vi "Pulse Measurement Panel.vi"(0 "RFmx Settings":T1={"Center Frequency (Hz)"=10000000000.0, "Measurement Bandwidth (Hz)"=80000000.0, "Reference Level (dBm)"=10.0, "RFmx De-embedding"={"RFmx Name"="5842_0", "RFmx Port"="", "Attenuation"={"Mode"=enum."Constant Attenuation", "Constant Attenuation"={"RFmx External Attenuation (dB)"=1.2}, "s2p File"={"RFmx S-Parameters Orientation"=24000, "RFmx Attenuation s2p Path Name"="", "RFmx Attenuation s2p File"=path ""}}}, "Acquisition Length (s)"=0.0} {"RFmx De-embedding"."Attenuation"."s2p File"."RFmx S-Parameters Orientation" items=["Port1 Towards DUT"=24000, "Port2 Towards DUT"=24001]; "RFmx De-embedding"."Attenuation"."Constant Attenuation"."RFmx External Attenuation (dB)" format="%.2f"; "Reference Level (dBm)" format="%.2f"; "Measurement Bandwidth (Hz)" format="%.3p"; "Center Frequency (Hz)" format="%.6p"}, 5 "RFSG settings":T3={"RFSG De-embedding"={"RFSG Name"="5842_0", "RFSG Port"="", "Attenuation"={"Mode"=enum."Constant Attenuation", "Contant Attenuation"={"RFSG External Attenuation (dB)"=2.0}, "s2p File"={"RFSG S-parameters Orientation"=24000, "RFSG Attenuation s2p Path Name"="", "RFSG s2p File Path"=path ""}}}, "Generation IQ Rate (S/s)"=0.0} {"RFSG De-embedding"."Attenuation"."s2p File"."RFSG S-parameters Orientation" items=["Port1 Towards DUT"=24000, "Port2 Towards DUT"=24001]; "RFSG De-embedding"."Attenuation"."Contant Attenuation"."RFSG External Attenuation (dB)" format="%.2f"}, 7 "Test Configuration":T5, 11 "error in":errorcluster) -> (3 "Per Pulse Results (Header Name)":string[](array[string]), 4 "TS Intrapulse Stability":dbl[][](array[numeric]), 6 "TS P2P Stability":dbl[][](array[numeric]), 8 "Per Pulse Results (for MP)":dbl[][](array[numeric])=[[-60.19434452056885, -48.23559761047363, -61.500163078308105, -61.676697731018066, -50.09932041168213, -61.2670373916626, -47.940940856933594, -60.594682693481445, -54.222588539123535, -68.17487716674805], [-51.47902011871338, -63.676371574401855, -49.32386875152588, -42.60602951049805, -41.78941249847412, -56.57611846923828, -67.04894065856934, -44.43309783935547, -53.89562129974365, -45.59821605682373], [-50.93127727508545, -48.11325550079346, -49.06841278076172, -42.55256652832031, -41.191606521606445, -55.30652046203613, -47.88793087005615, -44.32924270629883, -51.04572772979736, -45.574283599853516], [0.7774313706217917, 0.7743052754564207, 0.6733820768651879, 0.6972024148638998, 0.6739289285829677, 0.8012453172128895, 0.7789831746751243, 0.81331101938709, 0.6993593760935255, 0.7751122603266651], [-0.04818759954671978, -0.17045354969029822, -0.2937592841444876, -0.18006245433349588, -0.30206692305208827, -0.23840372056041464, -0.22733917807886903, -0.2726908323785403, -0.20409866605988866, -0.22706977878895118], [1.8971785430084185, 1.7078184861447125, 1.6125145446758244, 1.6429880662265446, 1.7003339064410368, 1.645767369340552, 1.8225724908268657, 1.500202053052531, 1.816586601520762, 1.7434164608706486], [9.902169056670972e-09, 1.0171003831640633e-08, 1.0087378671871648e-08, 1.0018839745468426e-08, 1.0021453073999283e-08, 9.937162678335199e-09, 1.0113660404718986e-08, 9.936247799288367e-09, 1.0029181489475149e-08, 1.0014254033422958e-08], [1.1747647026741224e-08, 0.00010001147191839247, 0.00020001407632828564, 0.0003000116995963527, 0.00040001415077715896, 0.0005000116894758734, 0.0006000140392077577, 0.000700011761394561, 0.0008000141195439436, 0.000900014054837663], [1.0266075038352937e-08, 1.0210194009332553e-08, 9.96602777140197e-09, 1.0195131948175912e-08, 1.0214687343427613e-08, 1.0248380139892106e-08, 1.003600972591812e-08, 1.0209683835273609e-08, 1.0208458229471944e-08, 1.0051256216333969e-08], [2.0016060941649103e-05, 0.00012001605265167608, 0.0002200186251165217, 0.0003200161244125173, 0.00042001858918951285, 0.0005200161200707459, 0.000620018587380489, 0.0007200160772447398, 0.0008200186061427676, 0.0009200186490169424], [1.9999915173664064e-05, 1.9999928162649538e-05, 1.9999979315091006e-05, 1.9999962883326592e-05, 1.9999940266618827e-05, 1.9999970715330443e-05, 1.9999948164994597e-05, 1.999989449659788e-05, 1.9999961878396942e-05, 2.0000044728873845e-05], [8.000006128542082e-05, 8.000009557087724e-05, 8.000003688745302e-05, 8.000002009960112e-05, 8.000005863752275e-05, 8.000001971001538e-05, 8.000010310677254e-05, 8.000006664992009e-05, 8.000000105017845e-05, nan], [19.999919881828227, 19.999923415962357, 19.999976074586076, 19.99996628673531, 19.99994048578986, 19.999972630258657, 19.999937910673005, 19.999902267256314, 19.99996929267048, nan], [9.999997645908488e-05, 0.00010000002373352679, 0.00010000001620254403, 9.999998298292771e-05, 9.999999890414157e-05, 9.999999042534582e-05, 0.00010000005127176714, 9.999996114651797e-05, 9.99999629285754e-05, nan]], 10 "TS Acquired Amplitude":dbl[][](array[numeric]), 15 "error out":errorcluster)   [LabVIEW 2023]
doc: "This example demonstrates the configuration of Pulse signal basic properties for measuring the stability properties of a pulse. This example enables traces to view the time domain stability and Pulse to Pulse Stability Traces ."
uses:
  Controls/RFmx Config - Pulse.ctl
  FPT Shared VIs/De-embedding/RFmx Config.ctl
  Controls/RFSG Config - Pulse.ctl
  FPT Shared VIs/De-embedding/RFsg Config.ctl
  Controls/Test Config - Pulse.ctl
panel:
  in  "Stop":bool
  in  "Configuration Tabs":enum32{"RFmx", "RFSG", "Test Configuration"}(tab)
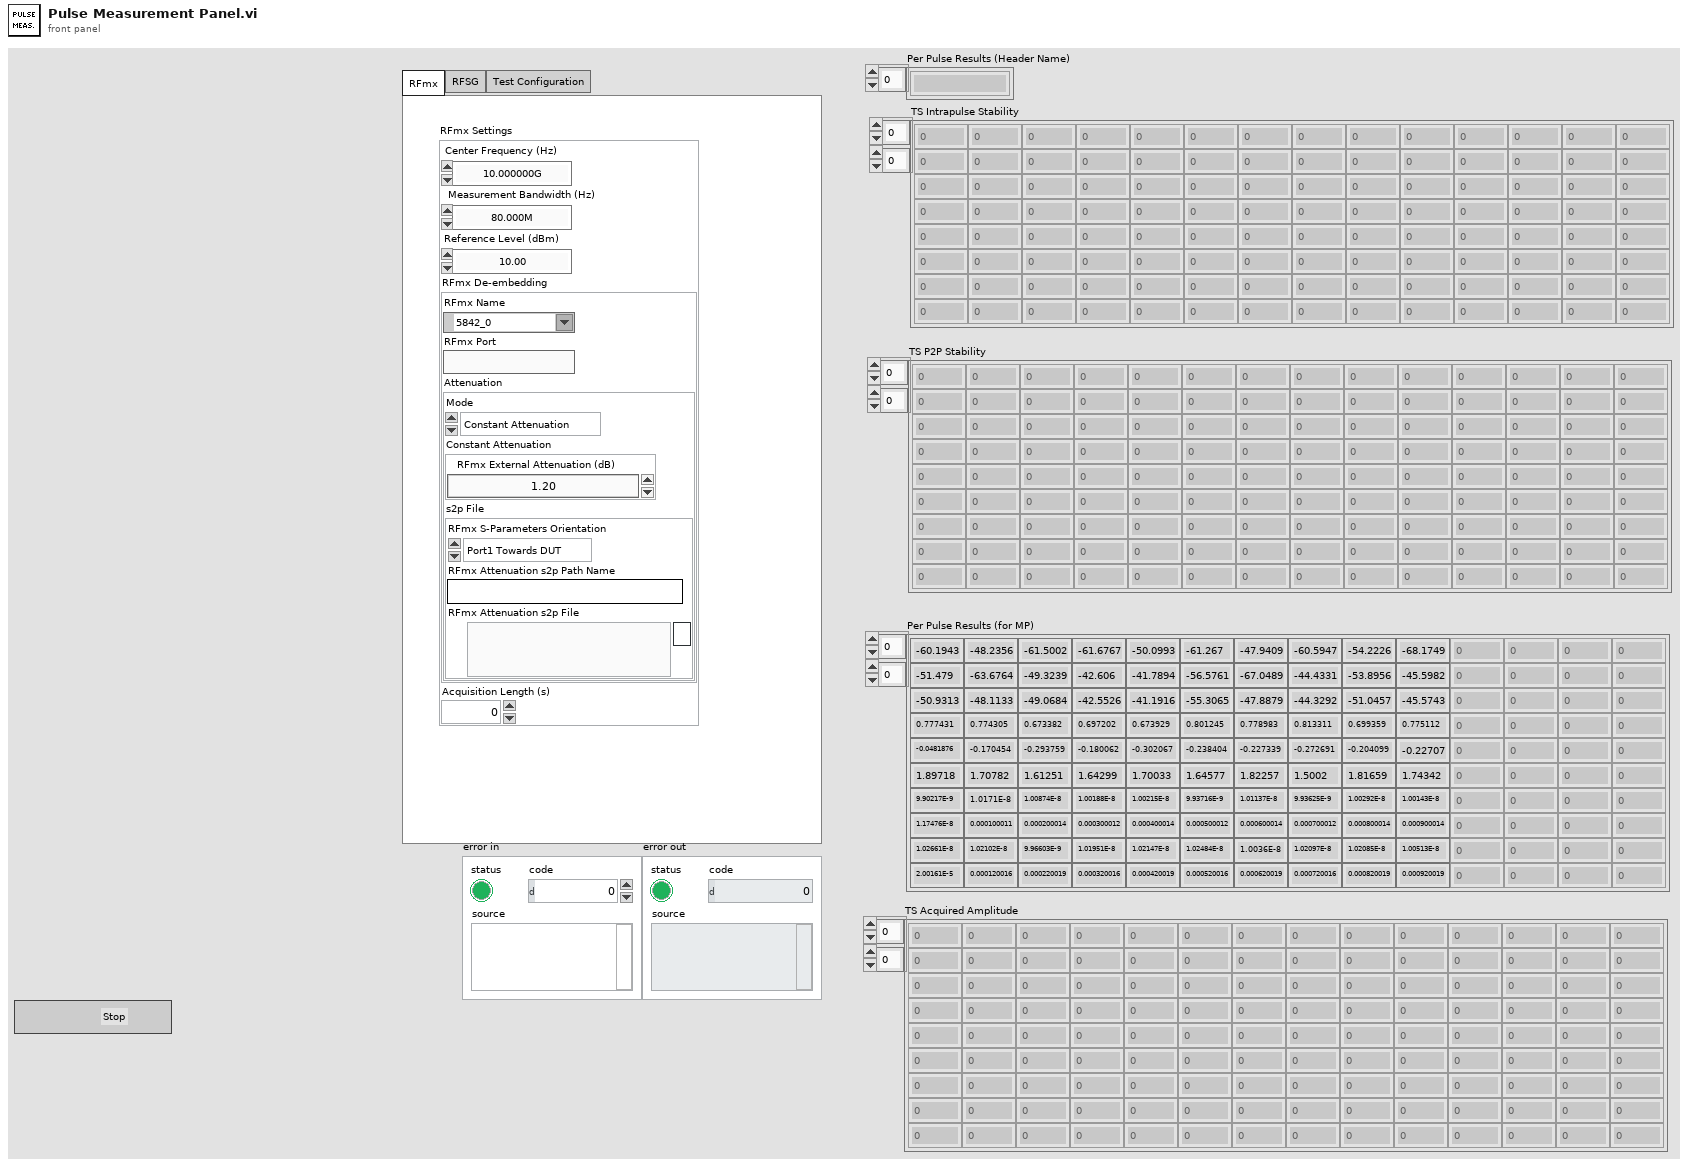
[diagram p1: front panel]
types:
  T1 = typedef "RFmx Config - Pulse.ctl" = cluster{"Center Frequency (Hz)":dbl, "Measurement Bandwidth (Hz)":dbl, "Reference Level (dBm)":dbl, "RFmx De-embedding":T2, "Acquisition Length (s)":dbl}
  T2 = typedef "RFmx Config.ctl" = cluster{"RFmx Name":refnum<k15>, "RFmx Port":string, "Attenuation":cluster{"Mode":enum32{"<None>", "Constant Attenuation", "s2p File"}, "Constant Attenuation":cluster{"RFmx External Attenuation (dB)":dbl}, "s2p File":cluster{"RFmx S-Parameters Orientation":i32, "RFmx Attenuation s2p Path Name":string, "RFmx Attenuation s2p File":path}}}
  T3 = typedef "RFSG Config - Pulse.ctl" = cluster{"RFSG De-embedding":T4, "Generation IQ Rate (S/s)":dbl}
  T4 = typedef "RFsg Config.ctl" = cluster{"RFSG Name":refnum<k15>, "RFSG Port":string, "Attenuation":cluster{"Mode":enum32{"<None>", "Constant Attenuation", "s2p File"}, "Contant Attenuation":cluster{"RFSG External Attenuation (dB)":dbl}, "s2p File":cluster{"RFSG S-parameters Orientation":i32, "RFSG Attenuation s2p Path Name":string, "RFSG s2p File Path":path}}}
  T5 = typedef "Test Config - Pulse.ctl" = cluster{"Pulse Configuration":cluster{"Power Level (dBm)":dbl, "Pulse Repetition Interval [PRI] (s)":dbl, "Pulse Width (s)":dbl, "Number of Pulses per Burst":u32}, "Pulse Stability":cluster{"Pulse Stability Meas Offset":i32, "Window Start (%)":dbl, "Window Stop (%)":dbl, "Window Step Size (%)":dbl, "Selected Pulse Trace":i32}, "Pulse Profile":cluster{"High Reference Level (%)":dbl, "Width Reference Level (%)":dbl, "Low Reference Level (%)":dbl}}
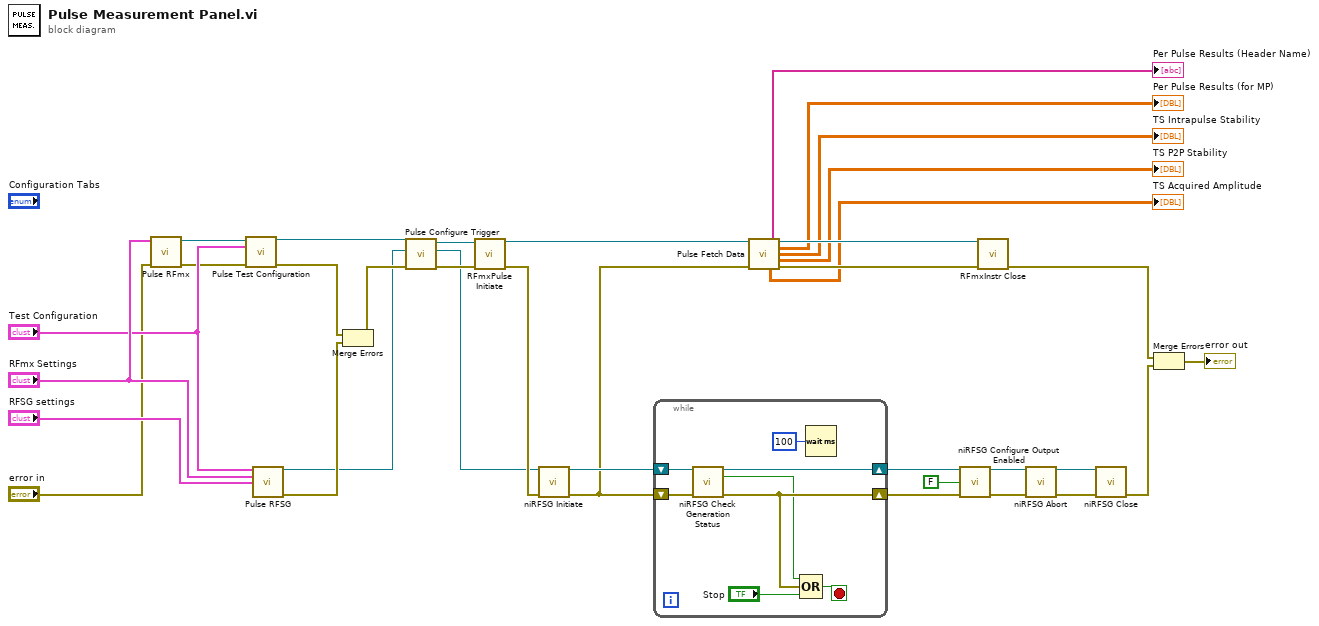
[diagram p0: block diagram]
diagram:
  n1 = call "Pulse RFmx.vi"("error in"="error in", "RFmx Settings"="RFmx Settings") -> ("error out"=w6:errorcluster, "RFmx session out"=w18:refnum<k21>)  [unwired: 8 in]
  n2 = call "Pulse Test Configuration.vi"("RFmx session in"=w18, "Test Configuration"="Test Configuration", "error in"=w6) -> ("RFmx session out"=w4:refnum<k21>, "error out"=w19:errorcluster)  [unwired: 11 in]
  n3 = call "Pulse RFSG.vi"("Test Configuration"="Test Configuration", "RFmx Settings"="RFmx Settings", "RFSG settings"="RFSG settings") -> ("RFSG session"=w2:refnum<k15>, "error out"=w20:errorcluster)  [unwired: 11 in]
  n4 = Merge Errors(w19, w20) -> (w24:errorcluster)
  n5 = call "Pulse Configure Trigger.vi"("error in"=w24, "RFSG session in"=w2, "RFmx session in"=w4) -> ("error out"=w5:errorcluster, "RFSG session out"=w1:refnum<k15>, "RFmx session out"=w3:refnum<k21>)  [unwired: 6 in]
  n6 = call <vilib>:"RFmxPulse Initiate.vi"("Instrument Handle In"=w3, "error in (no error)"=w5) -> ("Instrument Handle Out"=w33:refnum<k21>, "error out"=w28:errorcluster)  [unwired: 11 in, 1 out]
  n7 = call <instrlib>:"niRFSG Initiate.vi"("instrument handle"=w1, "error in"=w28) -> ("instrument handle out"=w32:refnum<k15>, "error out"=w27:errorcluster)  [unwired: 12 in]
  n8 = while {
    shift-right: [w42] -> w30
    shift-left: w32 -> [w43]
    shift-right: [w37] -> w29
    shift-left: w27 -> [w38]
    stop <- w41 stop-if-true
    n9 = call <instrlib>:"niRFSG Check Generation Status.vi"("instrument handle"=w43, "error in"=w38) -> ("instrument handle out"=w42:refnum<k15>, "done?"=w36:bool, "error out"=w37:errorcluster)  [unwired: 11 in]
    n10 = Compound Arithmetic op=OR(w36, w37, "Stop") -> (w41:bool)
    n11 = Wait (ms)(milliseconds to wait=u32 100) -> ()  [unwired: 1 out]
  }
  n12 = call "Pulse Fetch Data.vi"("RFmx Session in"=w33, "error in"=w27) -> ("Per Pulse Results (Header Name)"=→"Per Pulse Results (Header Name)":string[], "RFmx Session Out"=w35:refnum<k21>, "Per Pulse Results (for MP)"=→"Per Pulse Results (for MP)":dbl[][], "TS Intrapulse Stability"=→"TS Intrapulse Stability":dbl[][], "TS P2P Stability"=→"TS P2P Stability":dbl[][], "TS Acquired Amplitude"=→"TS Acquired Amplitude":dbl[][], "error out"=w34:errorcluster)  [unwired: 7 in]
  n13 = call <instrlib>:"niRFSG Configure Output Enabled.vi"("instrument handle"=w30, "output enabled"=FALSE ("output enable"), "error in"=w29) -> ("instrument handle out"=w22:refnum<k15>, "error out"=w21:errorcluster)  [unwired: 11 in]
  n14 = call <vilib>:"RFmxInstr Close.vi"("Instrument Handle In"=w35, "error in (no error)"=w34) -> ("error out"=w25:errorcluster)  [unwired: 13 in]
  n15 = call <instrlib>:"niRFSG Abort.vi"("instrument handle"=w22, "error in"=w21) -> ("instrument handle out"=w8:refnum<k15>, "error out"=w9:errorcluster)  [unwired: 12 in]
  n16 = call <instrlib>:"niRFSG Close.vi"("instrument handle"=w8, "error in"=w9) -> ("error out"=w23:errorcluster)  [unwired: 13 in]
  n17 = Merge Errors(w25, w23) -> (→"error out":errorcluster)
